vi "CONTROL CONVEYOR.vi"() -> ()   [LabVIEW 2018]
panel:
  in  "milliseconds to wait":u32
  in  "Boolean":bool
  out "Ring":u16(ring)
  in  "stop":bool
  in  "Slide 3":dbl(slide) scale=0.0..100.0
  in  "Slide 2":dbl(slide) scale=0.0..100.0
  out "Slide":cluster{dbl, dbl}(slide)={0.0, 0.9302325581395349} scale=0.0..100.0
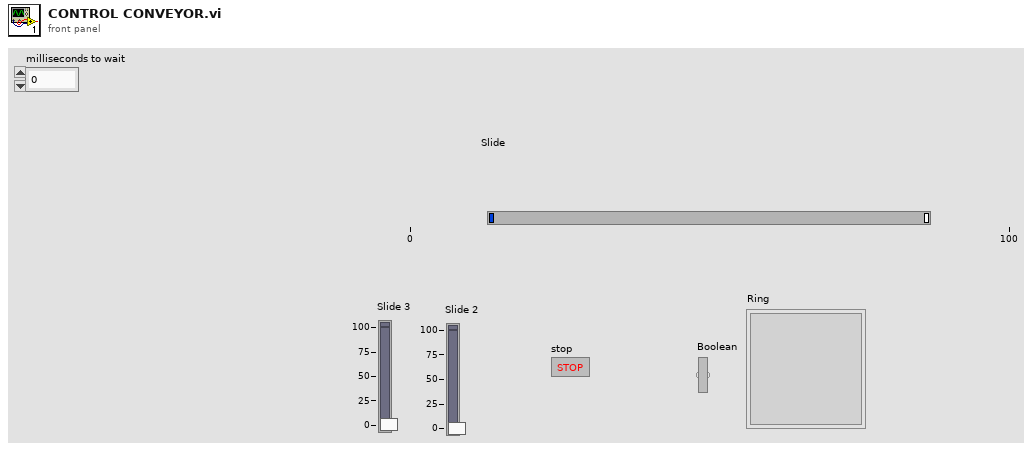
[diagram p1: front panel]
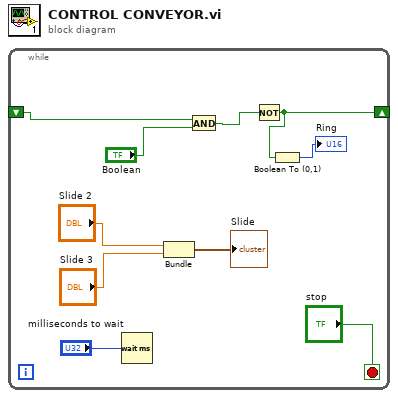
[diagram p0: block diagram]
diagram:
  n1 = while {
    shift-right: [w2] -> _
    shift-left: _ -> [w6]
    stop <- "stop" stop-if-true
    n2 = Wait (ms)(milliseconds to wait="milliseconds to wait") -> ()  [unwired: 1 out]
    n3 = Bundle("Slide 2"="Slide 2", "Slide 3"="Slide 3") -> (→"Slide":cluster{"Slide 2":dbl, "Slide 3":dbl})  [unwired: 1 in]
    n4 = And(x=w6, y="Boolean") -> (x .and. y?=w4:bool)
    n5 = Not(x=w4) -> (.not. x?=w2:bool)
    n6 = Boolean To (0,1)(Boolean=w2) -> (0, 1=→"Ring":i16)
  }
